vi "Pointyness screening.vi"(0 "Scan Loc":dbl[](array[numeric]), 2 "Feature Loc":dbl[](array[numeric]), 3 "Intensities":dbl[](array[numeric]), 4 "Peak\npointyness":dbl, 5 "2nd Derivatives":dbl[](array[numeric])) -> (6 "Scan Loc":dbl[](array[numeric]), 7 "Feature Loc":dbl[](array[numeric]), 8 "Intensities":dbl[](array[numeric]))   [LabVIEW 2014]
panel:
  out "size(s) 4":i32
  out "size(s) 3":i32
  out "size(s) 2":i32
  out "size(s)":i32
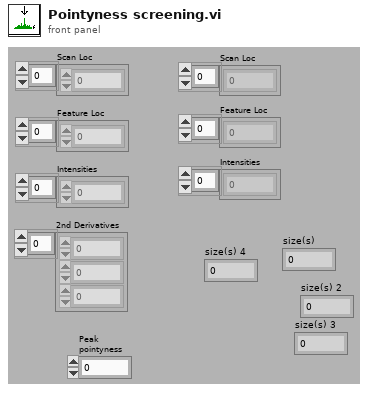
[diagram p1: front panel]
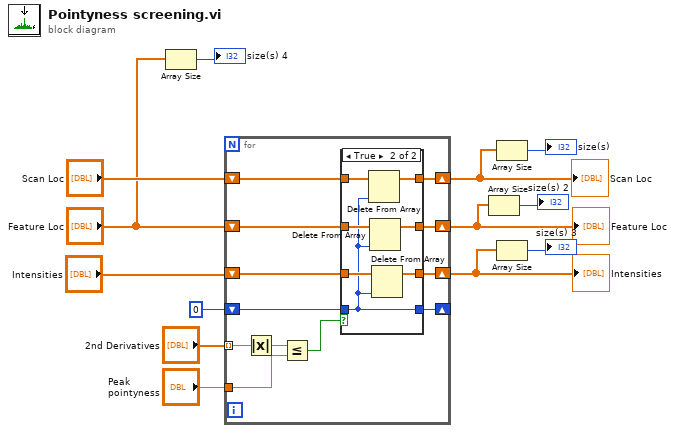
[diagram p0: block diagram]
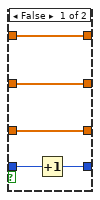
[diagram p2: hidden frame]
diagram:
  n1 = Array Size(array="Feature Loc") -> (size(s)=→"size(s) 4":i32)
  n2 = for {
    tunnel: "2nd Derivatives" -> [w16] mode=indexing
    shift-right: [w23] -> w8
    shift-left: "Scan Loc" -> [w25]
    shift-right: [w24] -> w5
    shift-left: "Feature Loc" -> [w22]
    shift-right: [w20] -> _
    shift-left: 0 -> [w21]
    shift-right: [w18] -> w3
    shift-left: "Intensities" -> [w19]
    tunnel: "Peak\npointyness" -> [w15]
    n3 = Absolute Value(x=w16) -> (abs(x)=w17:dbl)
    n4 = Less Or Equal?(x=w17, y=w15) -> (x <= y?=w14:bool)
    n5 = case shown="True" w14 {
      tunnel: w22 -> [w29 w34]
      tunnel: [w29 w35] -> w24
      tunnel: [w30 w37] -> w23
      tunnel: w25 -> [w30 w36]
      tunnel: w21 -> [w28 w31]
      tunnel: [w27 w31] -> w20
      tunnel: w19 -> [w26 w32]
      tunnel: [w26 w33] -> w18
      frame False {
        n6 = Increment(x=w28) -> (x+1=w27:i32)
      }
      frame True {
        n7 = Delete From Array(array=w36, index=w31) -> (array with subset deleted=w37:dbl[])  [unwired: 1 in, 1 out]
        n8 = Delete From Array(array=w34, index=w31) -> (array with subset deleted=w35:dbl[])  [unwired: 1 in, 1 out]
        n9 = Delete From Array(array=w32, index=w31) -> (array with subset deleted=w33:dbl[])  [unwired: 1 in, 1 out]
      }
    }
  }
  "Intensities" <- w3
  "Feature Loc" <- w5
  "Scan Loc" <- w8
  n10 = Array Size(array=w5) -> (size(s)=→"size(s) 2":i32)
  n11 = Array Size(array=w8) -> (size(s)=→"size(s)":i32)
  n12 = Array Size(array=w3) -> (size(s)=→"size(s) 3":i32)
